vi "Untitled 4 (SubVI).vi"(10 "Array":u16[][](array[numeric]), 11 "Array 2":u16[](array[numeric])) -> (1 "Waveform Chart":dbl(graph), 2 "Temperature(°C)":dbl, 3 "Numeric":dbl)   [LabVIEW 2016]
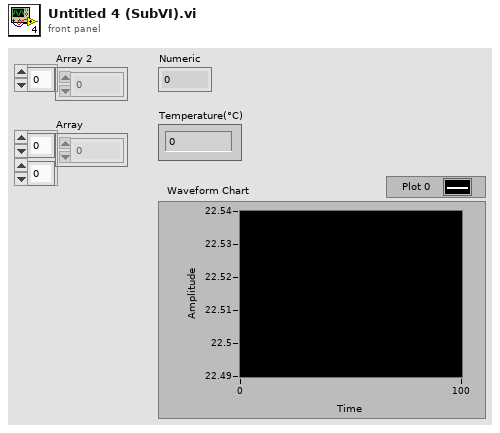
[diagram p1: front panel]
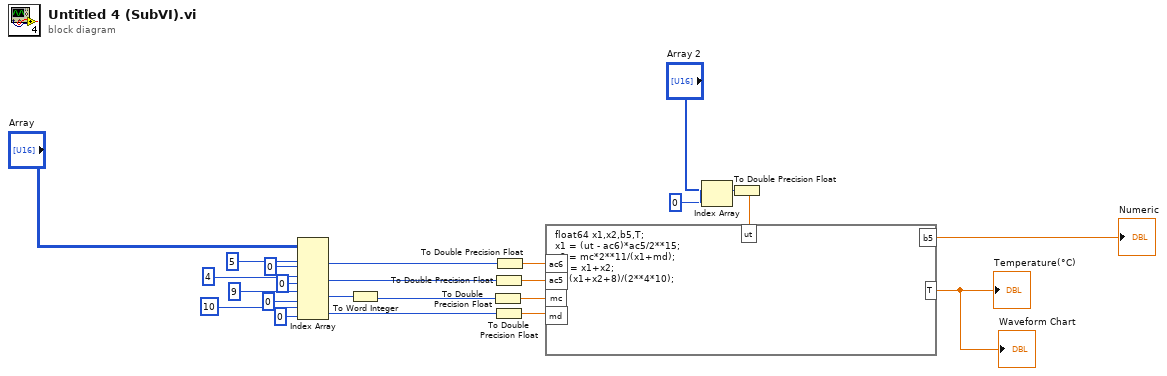
[diagram p0: block diagram]
diagram:
  n1 = Index Array(array="Array", index (row) #1=5 ("index (row)"), index (col) #1=0 ("disabled index (col)"), index (row) #2=4, index (col) #2=0 ("disabled index (col)"), index (row) #3=9 ("index (row)"), index (col) #3=0 ("disabled index (col)"), index (row) #4=10, index (col) #4=0 ("disabled index (col)")) -> (element #1=w6:u16, element #2=w7:u16, element #3=w11:u16, element #4=w8:u16)
  n2 = To Word Integer(number=w11) -> (16bit integer=w12:i16)
  n3 = To Double Precision Float(number=w12) -> (double precision float=w19:dbl)
  n4 = To Double Precision Float(number=w7) -> (double precision float=w18:dbl)
  n5 = To Double Precision Float(number=w8) -> (double precision float=w20:dbl)
  n6 = To Double Precision Float(number=w6) -> (double precision float=w17:dbl)
  n7 = Index Array(array="Array 2", index=0) -> (element=w15:u16)
  n8 = To Double Precision Float(number=w15) -> (double precision float=w16:dbl)
  n9 = formula code="float64 x1,x2,b5,T;\nx1 = (ut - ac6)*ac5/2**15;\nx2 = mc*2**11/(x1+md);\nb5 = x1+x2;\nT=(x1+x2+8)/(2**4*10);"("mc"=w19, "md"=w20, "ac5"=w18, "ac6"=w17, "ut"=w16) -> ("T"=→"Temperature(°C)" →"Waveform Chart":dbl, "b5"=→"Numeric":dbl)
